vi "camera kive feed trial.vi"() -> ()   [LabVIEW 2025]
uses:
  D:/Projects/BOCLE/WO 2479/v01/MAIN SCREEN SUPPORT VI's/CAMERA LIVE FEED ENUM.ctl
  c9f947c2-6258-4522-b007-cc7728108fad.vi
  7b5bd523-c89b-4302-84cf-76e6829f20d7.vi
  720e3916-1574-49a6-b2fa-09813ce45a3a.vi
  53088a8a-16f5-4225-8c3d-04506246f421.vi
  a160c775-0709-4436-9dd3-45acf388d4d1.vi
  c7a23adb-69d7-42db-ae3b-33f4a2a04bd7.vi
  acb06eee-55f0-46c0-9ea2-f9dce46418b0.vi
  f58cf036-ef32-4f52-94af-0e7fd84df475.vi
panel:
  out "error out":errorcluster
  in  "stop":bool
  in  "Combo Box - Autocomplete":string(combo)
  out "data out":string
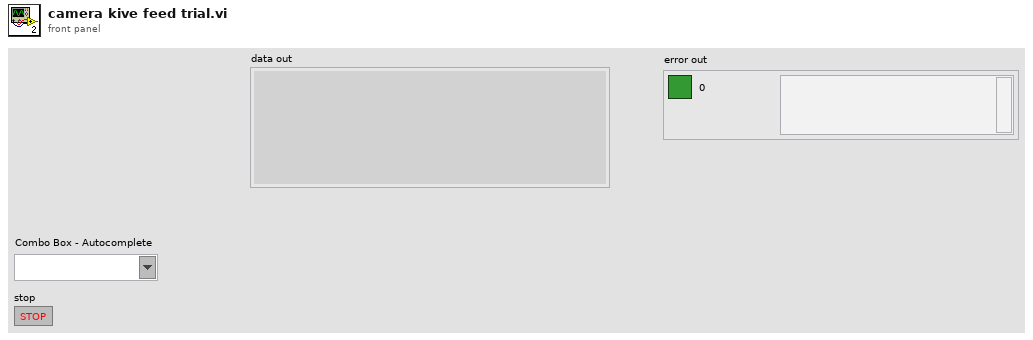
[diagram p1: front panel]
types:
  T1 = typedef "CAMERA LIVE FEED ENUM.ctl" = enum16{"OPEN EXE", "INIT", "READ", "CAMERA CONNECT", "CAMERA START", "CAMERA STOP", "CAMERA GRAY", "CAMERA RGB", "CAMERA MINIMIZE", "CAMERA CLOSE", "CAMERA MODE LIST", "CAMERA MODE SET", "CAMERA RESTORE", "CAMERA SAVE", "CLOSE"}
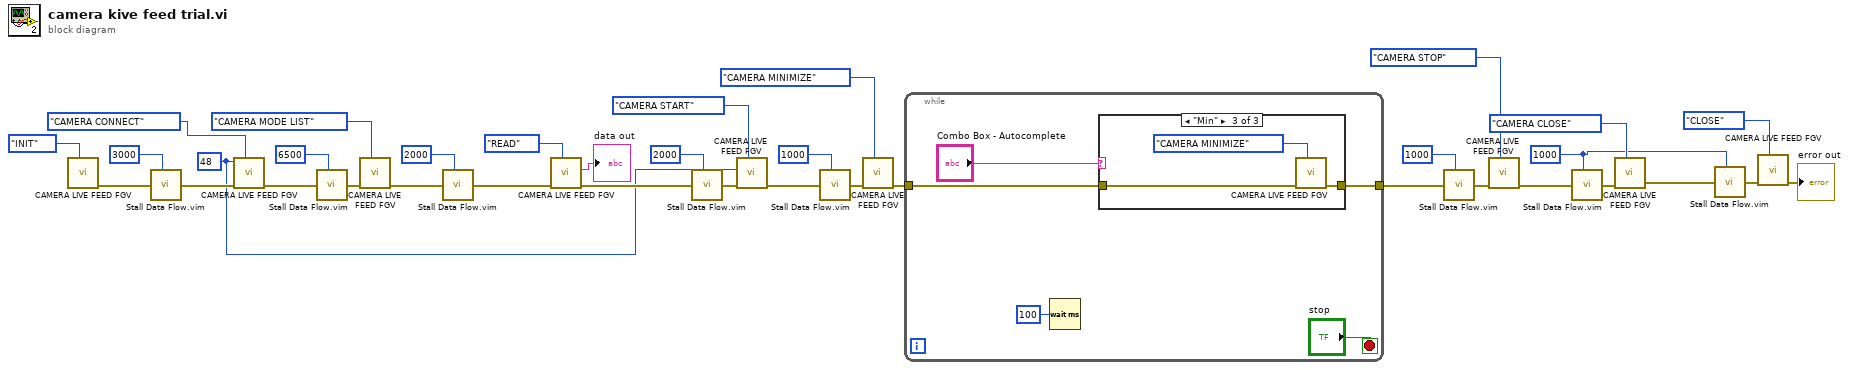
[diagram p0: block diagram]
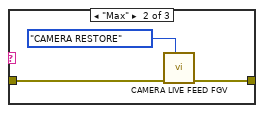
[diagram p3: hidden frame]
diagram:
  w2 = u32 1000 ("milliseconds to wait")
  w6 = u8 48 ("CAMERA PORT")
  n1 = call "CAMERA LIVE FEED FGV.vi"("Enum - Menu"=CAMERA_LIVE_FEED_ENUM."INIT") -> ("error out"=w35:errorcluster)  [unwired: 9 in, 1 out]
  n2 = call "Stall Data Flow.vim"("value in"=w35, "milliseconds to wait"=u32 3000) -> ("value out"=w34:errorcluster)  [unwired: 1 out]
  n3 = call "CAMERA LIVE FEED FGV.vi"("Enum - Menu"=CAMERA_LIVE_FEED_ENUM."CAMERA CONNECT", "error in (no error)"=w34, "CAMERA PORT"=w6) -> ("error out"=w32:errorcluster)  [unwired: 7 in, 1 out]
  n4 = call "Stall Data Flow.vim"("value in"=w32, "milliseconds to wait"=u32 6500) -> ("value out"=w30:errorcluster)  [unwired: 1 out]
  n5 = call "CAMERA LIVE FEED FGV.vi"("Enum - Menu"=CAMERA_LIVE_FEED_ENUM."CAMERA MODE LIST", "error in (no error)"=w30) -> ("error out"=w27:errorcluster)  [unwired: 8 in, 1 out]
  n6 = call "Stall Data Flow.vim"("value in"=w27, "milliseconds to wait"=u32 2000) -> ("value out"=w28:errorcluster)  [unwired: 1 out]
  n7 = call "CAMERA LIVE FEED FGV.vi"("Enum - Menu"=CAMERA_LIVE_FEED_ENUM."READ", "error in (no error)"=w28) -> ("error out"=w24:errorcluster, "data out"=→"data out":string)  [unwired: 8 in]
  n8 = call "Stall Data Flow.vim"("value in"=w24, "milliseconds to wait"=u32 2000) -> ("value out"=w20:errorcluster)  [unwired: 1 out]
  n9 = call "CAMERA LIVE FEED FGV.vi"("Enum - Menu"=CAMERA_LIVE_FEED_ENUM."CAMERA START", "error in (no error)"=w20, "CAMERA MODE"=w6) -> ("error out"=w19:errorcluster)  [unwired: 7 in, 1 out]
  n10 = call "Stall Data Flow.vim"("value in"=w19, "milliseconds to wait"=u32 1000) -> ("value out"=w17:errorcluster)  [unwired: 1 out]
  n11 = call "CAMERA LIVE FEED FGV.vi"("Enum - Menu"=CAMERA_LIVE_FEED_ENUM."CAMERA MINIMIZE", "error in (no error)"=w17) -> ("error out"=w15:errorcluster)  [unwired: 8 in, 1 out]
  n12 = while {
    tunnel: w15 -> [w40]
    tunnel: [w39] -> w10
    stop <- "stop" stop-if-true
    n13 = Wait (ms)(milliseconds to wait=u32 100) -> ()  [unwired: 1 out]
    n14 = case shown="\"Min\"" "Combo Box - Autocomplete" {
      tunnel: w40 -> [w42 w44 w47]
      tunnel: [w42 w43 w46] -> w39
      frame "No Task", Default {
      }
      frame "Max" {
        n15 = call "CAMERA LIVE FEED FGV.vi"("Enum - Menu"=CAMERA_LIVE_FEED_ENUM."CAMERA RESTORE", "error in (no error)"=w44) -> ("error out"=w43:errorcluster)  [unwired: 8 in, 1 out]
      }
      frame "Min" {
        n16 = call "CAMERA LIVE FEED FGV.vi"("Enum - Menu"=CAMERA_LIVE_FEED_ENUM."CAMERA MINIMIZE", "error in (no error)"=w47) -> ("error out"=w46:errorcluster)  [unwired: 8 in, 1 out]
      }
    }
  }
  n17 = call "Stall Data Flow.vim"("value in"=w10, "milliseconds to wait"=u32 1000) -> ("value out"=w11:errorcluster)  [unwired: 1 out]
  n18 = call "CAMERA LIVE FEED FGV.vi"("Enum - Menu"=CAMERA_LIVE_FEED_ENUM."CAMERA STOP", "error in (no error)"=w11) -> ("error out"=w7:errorcluster)  [unwired: 8 in, 1 out]
  n19 = call "Stall Data Flow.vim"("value in"=w7, "milliseconds to wait"=w2) -> ("value out"=w9:errorcluster)  [unwired: 1 out]
  n20 = call "CAMERA LIVE FEED FGV.vi"("Enum - Menu"=CAMERA_LIVE_FEED_ENUM."CAMERA CLOSE", "error in (no error)"=w9) -> ("error out"=w3:errorcluster)  [unwired: 8 in, 1 out]
  n21 = call "Stall Data Flow.vim"("value in"=w3, "milliseconds to wait"=w2) -> ("value out"=w4:errorcluster)  [unwired: 1 out]
  n22 = call "CAMERA LIVE FEED FGV.vi"("Enum - Menu"=CAMERA_LIVE_FEED_ENUM."CLOSE", "error in (no error)"=w4) -> ("error out"=→"error out":errorcluster)  [unwired: 8 in, 1 out]
